vi "About.vi"(8 "error in (no error)":errorcluster, 10 "Items Edited":u32, 11 "Calling VI in":refnum<vi>) -> (0 "error out":errorcluster)   [LabVIEW 2020, in "VI Properties Editor.lvlib"]
doc: "Displays a window that shows various information about the tool."
uses:
  VI Properties Editor.lvlib
panel:
  out "Usage Info":string="Total number of items edited: #"
  out "Version Info":string="version #.#.#.# - Month DD, YYYY"
  # "VI Properties Editor"
  # "by Andrew Casalenuovo"
  # "VIPM Package: https://www.vipm.io/package/redhawk_lib_vi_properties_editor/"
  # "GitHub Repository: https://github.com/FireFist-Redhawk/VI-Properties-Editor"
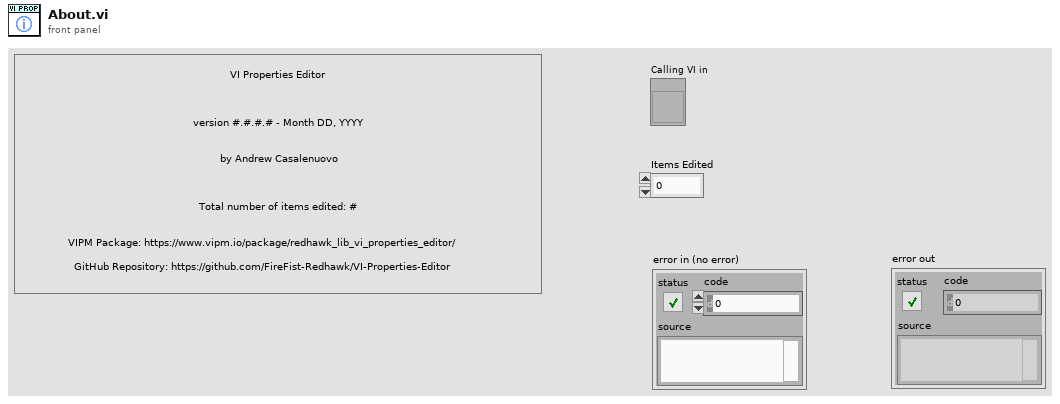
[diagram p1: front panel]
types:
  T1 = enum32{"Invalid", "Standard", "Closed", "Hidden", "Minimized", "Maximized"}
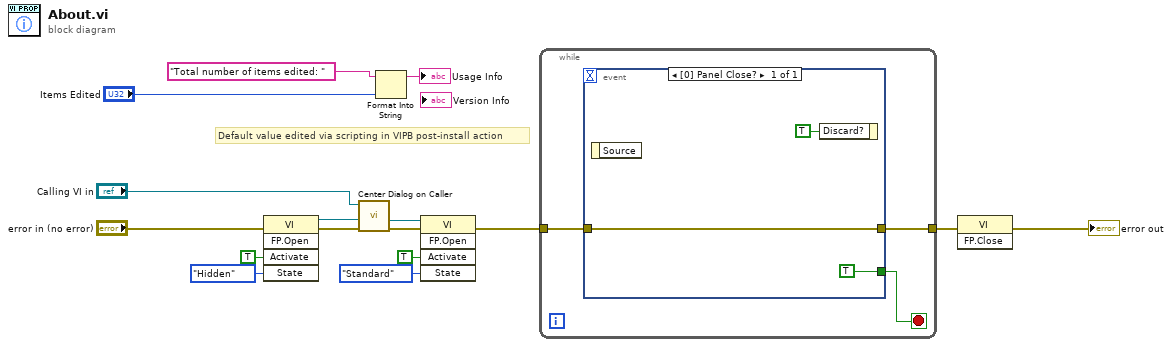
[diagram p0: block diagram]
diagram:
  # "Default value edited via scripting in VIPB post-install action"
  n1 = invoke class="VI" method="FP.Open"(error in="error in (no error)", "Activate"=TRUE ("Activate?"), "State"=T1."Hidden") -> (reference out=w8:refnum<vi>, error out=w10:errorcluster)  [unwired: 2 in, 3 out]
  n2 = call "Center Dialog on Caller.vi"("error in (no error)"=w10, "Dialog VI"=w8, "Calling VI in"="Calling VI in") -> ("error out"=w5:errorcluster, "Dialog VI out"=w4:refnum<vi>)  [unwired: 7 in]
  n3 = Format Into String(initial string="Total number of items edited: ", "Items Edited") -> (resulting string=→"Usage Info":string)  [unwired: 2 in, 1 out]
  n4 = invoke class="VI" method="FP.Open"(reference=w4, error in=w5, "Activate"=TRUE ("Activate?"), "State"=T1."Standard") -> (error out=w14:errorcluster)  [unwired: 1 in, 4 out]
  n5 = while {
    tunnel: [w18] -> w16
    tunnel: w14 -> [w17]
    stop <- w19 stop-if-true
    n6 = event shown="[0] Panel Close?" {
      selector: _ -> [_]
      dyn-events: _ -> [_]
      timeout: _ -> [_]
      tunnel: [TRUE] -> w19
      tunnel: [w20] -> w18
      tunnel: w17 -> [w20]
      event Panel Close? {
        n7 = event-data() -> ()  [unwired: 1 in, 1 out]
        n8 = event-data("Discard?"=TRUE) -> ()  [unwired: 1 in, 1 out]
      }
    }
  }
  n9 = invoke class="VI" method="FP.Close"(error in=w16) -> (error out=→"error out":errorcluster)  [unwired: 2 in, 2 out]
